vi "Close TDMS Log File.vi"(8 "error in (no error)":errorcluster, 11 "TDMS Log File in":refnum<class "TDMS Log File.lvclass">) -> (0 "error out":errorcluster, 3 "File Path":path)   [LabVIEW 2015, in "TDMS Log File.lvclass"]
uses:
  TDMS Log File.lvclass
  TDMS Log File.lvclass/TDMS Log File.ctl
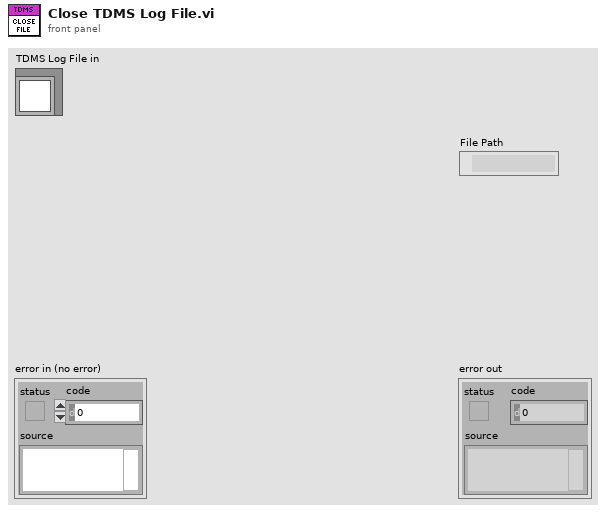
[diagram p1: front panel]
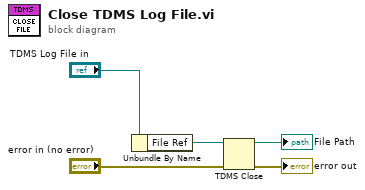
[diagram p0: block diagram]
diagram:
  n1 = Unbundle By Name("TDMS Log File in") -> ("File Ref"=w3:refnum<k34>)
  n2 = TDMS Close(8:"error in (no error)", 11:w3) -> (0:→"error out":errorcluster, 3:→"File Path":path)
